vi "Get_AC_IR_Config.vi"(8 "error in (no error)":errorcluster caption="错误输入（无错误）", 11 "组合框":string(combo)) -> (0 "error out":errorcluster, 2 "OutData":string[](array[string]), 3 "添加的路径":path)   [LabVIEW 2018]
uses:
  Global.vi
  <vilib>/Utility/config.llb/Read Key (String).vi
  <vilib>/Utility/config.llb/NI_LVConfig.lvlib
panel:
  out "数组":string[](array[string])
  out "元素":string
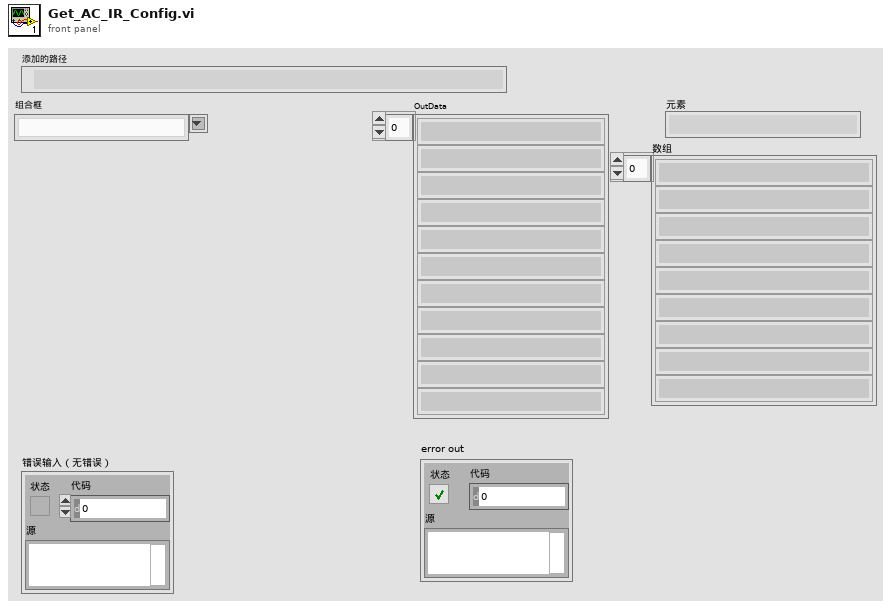
[diagram p1: front panel]
types:
  T1 = typedef "NI_LVConfig.lvlib/Config Data RefNum.ctl" = refnum<k1>
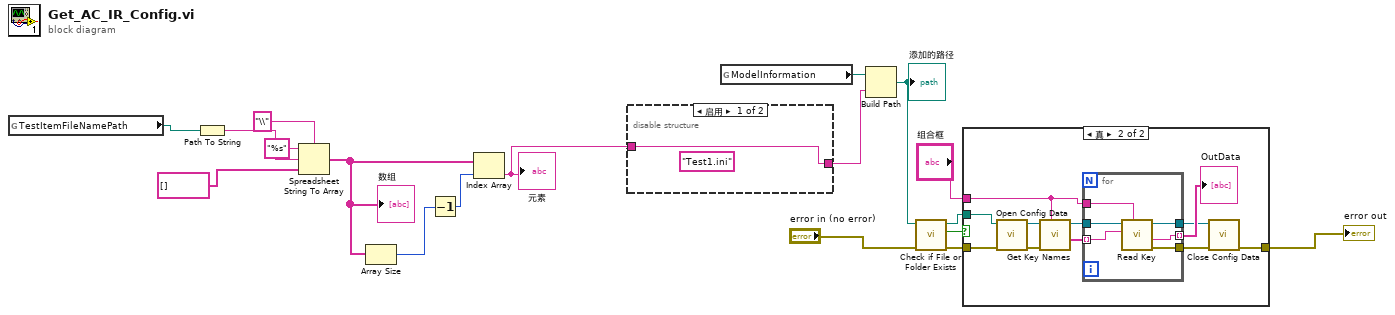
[diagram p0: block diagram]
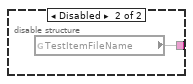
[diagram p2: hidden frame]
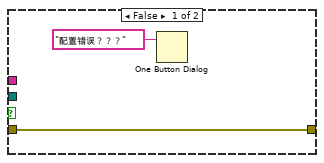
[diagram p3: hidden frame]
diagram:
  n1 = global read "Global.vi" "TestItemFileNamePath"() -> (w18:path)
  n2 = Path To String(path=w18) -> (string=w16:string)
  n3 = Spreadsheet String To Array(delimiter (Tab)="\\" ("分隔符(Tab)"), format string="%s" ("格式字符串"), spreadsheet string=w16, array type (2D Dbl)=string[] []) -> (array=w14:string[])
  "数组" <- w14
  n4 = Array Size(array=w14) -> (size(s)=w13:i32)
  n5 = Decrement(x=w13) -> (x-1=w11:i32)
  n6 = Index Array(array=w14, index=w11) -> (element=w1:string)
  "元素" <- w1
  n7 = disable-structure shown="启用" {
    disable-tunnel: [w19 w20] -> w6
    disable-tunnel: w1 -> [w19 _]
    frame Enabled {
      (unwired) "Test1.ini" ("名称或相对路径")
    }
    frame Disabled {
      n8 = global read "Global.vi" "TestItemFileName"() -> (w20)
    }
  }
  n9 = global read "Global.vi" "ModelInformation"() -> (w5:path)
  n10 = Build Path(base path=w5, name or relative path=w6) -> (appended path=w4:path)
  "添加的路径" <- w4
  n11 = call <vilib>:"Check if File or Folder Exists.vi"("error in (no error)"="error in (no error)", "path"=w4) -> ("error out"=w8:errorcluster, "file or folder exists?"=w10:bool, "dup path"=w9:path)  [unwired: 7 in]
  n12 = case shown="真" w10 {
    tunnel: w9 -> [_ w33]
    tunnel: w8 -> [w21 w32]
    tunnel: "组合框" -> [_ w26]
    tunnel: [w21 w23] -> w3
    frame False {
      n13 = One Button Dialog(message="配置错误？？？" ("消息")) -> ()  [unwired: 1 in, 1 out]
    }
    frame True {
      n14 = call <vilib>:"Open Config Data.vi"("error in (no error)"=w32, "configuration file path"=w33) -> ("error out"=w30:errorcluster, "refnum"=w31:T1)  [unwired: 7 in, 1 out]
      n15 = call <vilib>:"Get Key Names.vi"("section"=w26, "error in (no error)"=w30, "refnum"=w31) -> ("key names"=w28:string[], "refnum out"=w29:T1)  [unwired: 5 in, 2 out]
      n16 = for {
        tunnel: w29 -> [w39]
        tunnel: w28 -> [w38] mode=indexing
        tunnel: [w37] -> w27 mode=indexing
        tunnel: w26 -> [w36]
        tunnel: [w35] -> w25
        tunnel: [w34] -> w24
        n17 = call-poly <vilib>:"Read Key.vi"("section"=w36, "key"=w38, "refnum"=w39) -> ("error out"=w34:errorcluster, "value"=w37:string, "refnum out"=w35:T1)  [unwired: 5 in, 1 out]
      }
      "OutData" <- w27
      n18 = call <vilib>:"Close Config Data.vi"("error in (no error)"=w24, "refnum"=w25) -> ("error out"=w23:errorcluster)  [unwired: 8 in, 1 out]
    }
  }
  "error out" <- w3
